vi "Write Time Stamp.vi"(8 "Error In":errorcluster, 10 "Time Stamp":timestamp format="%<%x %.3X>T", 11 "Add Value with TS Msg":refnum<class "Add Value with TS Msg.lvclass">) -> (0 "Error Out":errorcluster, 3 "Add Value with TS Msg":refnum<class "Add Value with TS Msg.lvclass">)   [LabVIEW 2019, in "BNT_XtGraph.lvlib" / "Add Value with TS Msg.lvclass"]
uses:
  Add Value with TS Msg.lvclass
  Add Value with TS Msg.lvclass/Add Value with TS Msg.ctl
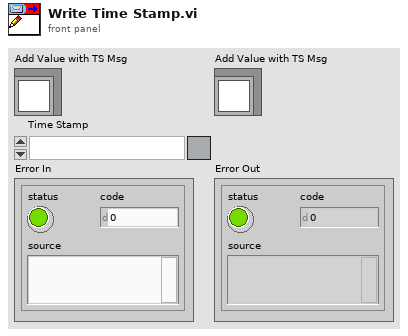
[diagram p1: front panel]
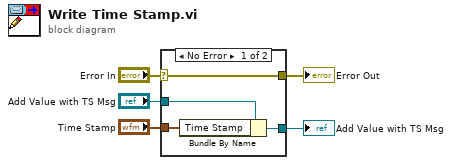
[diagram p0: block diagram]
diagram:
  n1 = case shown="No Error" "Error In" {
    selector: "Error In" -> [w9 w10]
    tunnel: [w9 w10] -> w5
    tunnel: [w7 w11] -> w3
    tunnel: "Add Value with TS Msg" -> [w8 w11]
    tunnel: "Time Stamp" -> [w6 _]
    frame No Error {
      n2 = Bundle By Name(cluster=w8, "Time Stamp"=w6) -> (w7:refnum<class "Add Value with TS Msg.lvclass">)
    }
    frame Error {
    }
  }
  "Add Value with TS Msg" <- w3
  "Error Out" <- w5
